vi "DELETE Number of Samples [Slope Calibration].vi"   [LabVIEW 2013]
uses:
  Action.ctl
  Slope Calibration Inputs FGV Selector.ctl
types:
  T1 = typedef "Slope Calibration Inputs FGV Selector.ctl" = enum16{"Number of Samples", "Ramp Rate", "Z Scan Size"}
  T2 = typedef "Action.ctl" = enum16{"GET", "PUT", "DELETE"}
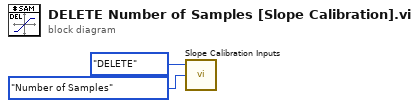
[diagram p0: block diagram]
diagram:
  n1 = call "Slope Calibration Inputs.vi"("Slope Calibration Inputs FGV Selector"=Slope_Calibration_Inputs_FGV_Selector."Number of Samples", "Action"=Action."DELETE") -> ()  [unwired: 1 in, 1 out]
